vi "FailureDescription.vi"(8 "error in (no error)":errorcluster, 10 "Actual":variant, 11 "ErrorMessageContains in":refnum<class "ErrorMessageContains.lvclass">) -> (0 "error out":errorcluster, 2 "Failure Description":string, 3 "ErrorMessageContains out":refnum<class "ErrorMessageContains.lvclass">)   [LabVIEW 2017, in "Transparent Assertions.lvlib" / "ErrorMessageContains.lvclass"]
doc: "Return the second part of the scentence \"Failed asserting that ...\""
uses:
  ErrorMessageContains.lvclass
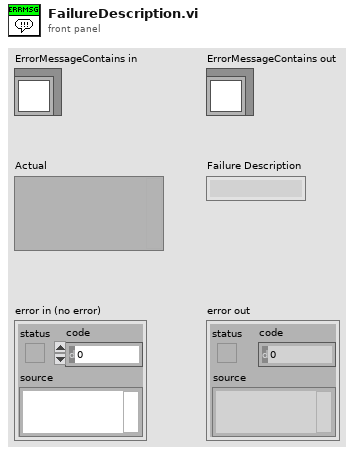
[diagram p1: front panel]
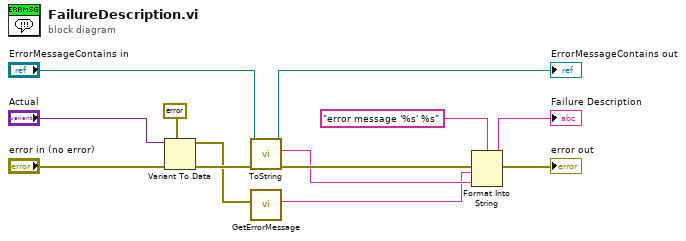
[diagram p0: block diagram]
diagram:
  n1 = Variant To Data(error in="error in (no error)", type=errorcluster {"status"=FALSE, "code"=0, "source"=""} ("error constant"), Variant="Actual") -> (data=w2:errorcluster, error out=w13:errorcluster)
  n2 = call-dynamic "ToString.vi"("error in (no error)"=w13, "ErrorMessageContains in"="ErrorMessageContains in") -> ("error out"=w11:errorcluster, "String"=w9:string, "ErrorMessageContains out"=→"ErrorMessageContains out":refnum<class "ErrorMessageContains.lvclass">)  [unwired: 7 in]
  n3 = call "GetErrorMessage.vi"("error in (no error)"=w2) -> ("Error Message"=w1:string)  [unwired: 10 in]
  n4 = Format Into String(format string="error message '%s' %s", error in=w11, w1, w9) -> (resulting string=→"Failure Description":string, error out=→"error out":errorcluster)  [unwired: 1 in]
